vi "LineFollower.vi"() -> ()   [LabVIEW 2019]
uses:
  <vilib>/addons/Fuzzy Logic/TypeDefs/FL System.ctl
  <vilib>/addons/Fuzzy Logic/TypeDefs/FL Variable.ctl
  <vilib>/addons/Fuzzy Logic/TypeDefs/FL Membership Function.ctl
  <vilib>/addons/Fuzzy Logic/TypeDefs/FL Membership Function Shape.ctl
  <vilib>/addons/Fuzzy Logic/TypeDefs/FL Rule.ctl
  <vilib>/addons/Fuzzy Logic/TypeDefs/FL Antecedent.ctl
  <vilib>/addons/Fuzzy Logic/TypeDefs/FL Modifier.ctl
  <vilib>/addons/Fuzzy Logic/TypeDefs/FL Antecedent Connective.ctl
  <vilib>/addons/Fuzzy Logic/TypeDefs/FL Consequent.ctl
  <vilib>/addons/Fuzzy Logic/TypeDefs/FL Consequent Implication.ctl
  <vilib>/addons/Fuzzy Logic/TypeDefs/FL Defuzzification.ctl
  <vilib>/addons/Fuzzy Logic/TypeDefs/FL Interpolating polynomials.ctl
  <vilib>/myRIO/Instrument Drivers/Onboard IO/AI/typedefs/AI Reference.ctl
  <vilib>/myRIO/Common/Instrument Driver Framework/Utilities/typedefs/myRIO Generic Hardware Reference.ctl
  <vilib>/myRIO/Common/Instrument Driver Framework/Utilities/typedefs/Hardware Version Enum.ctl
  <vilib>/myRIO/Common/Instrument Driver Framework/Utilities/typedefs/myRIO v1.0 Reference.ctl
  <vilib>/myRIO/Common/Instrument Driver Framework/Utilities/typedefs/Generic FPGA Reference.ctl
  <vilib>/myRIO/Common/Instrument Driver Framework/myRIO v1.0/AI/typedefs/AI Channels List.ctl
  <vilib>/myRIO/Common/Instrument Driver Framework/myRIO v1.0/AI/typedefs/AI Channels Enum.ctl
  <vilib>/myRIO/Common/Instrument Driver Framework/Utilities/typedefs/Analog Scaling Constants List.ctl
  <vilib>/myRIO/Common/Instrument Driver Framework/Utilities/typedefs/Analog Scaling Constants.ctl
  <vilib>/userdefined/High Color/nirio_resource_hc.ctl
  <vilib>/myRIO/Common/Instrument Driver Framework/Utilities/vis/Is FPGA Ref Available.vi
  <vilib>/myRIO/Common/Instrument Driver Framework/myRIO v1.0/AI/vis/myRIO v1.1 Open AI.vi
  <vilib>/myRIO/Instrument Drivers/Onboard IO/AI/vis/Read.vi
  <vilib>/myRIO/Common/Instrument Driver Framework/Utilities/vis/Validate Channels.vi
  <vilib>/myRIO/Common/Instrument Driver Framework/myRIO v1.0/AI/vis/myRIO v1.0 Reserve AI.vi
  <vilib>/myRIO/Common/Instrument Driver Framework/myRIO v1.0/AI/vis/myRIO v1.0 Build MUX Configuration AI.vi
  <vilib>/myRIO/Common/Instrument Driver Framework/myRIO v1.0/Resource Manager/vis/myRIO v1.0 Reserve Channel List.vi
  <vilib>/myRIO/Common/Instrument Driver Framework/myRIO v1.0/Resource Manager/vis/myRIO v1.0 Reserve Channel.vi
  <vilib>/myRIO/Common/Instrument Driver Framework/myRIO v1.0/Resource Manager/vis/myRIO v1.0 Unreserve Channel.vi
  <vilib>/myRIO/Common/Instrument Driver Framework/myRIO v1.0/Resource Manager/vis/myRIO v1.0 Build Mutex Name.vi
  <vilib>/Utility/VariantDataType/GetNumericInfo.vi
  <vilib>/Utility/error.llb/Error Cluster From Error Code.vi
  <vilib>/myRIO/Common/Instrument Driver Framework/myRIO v1.0/myRIO v1.1 Open.vi
  <vilib>/myRIO/Common/Instrument Driver Framework/myRIO v1.0/AI/vis/myRIO v1.0 Get Scaling Constants AI.vi
  <vilib>/myRIO/Common/Instrument Driver Framework/Utilities/vis/IO Manager.vi
  <vilib>/myRIO/Common/Instrument Driver Framework/Utilities/vis/Configuration Manager.vi
  <vilib>/myRIO/Common/Instrument Driver Framework/myRIO v1.0/myRIO v1.0 Close.vi
  <vilib>/myRIO/Common/Instrument Driver Framework/myRIO v1.0/AI/vis/myRIO v1.0 Read AI.vi
  <vilib>/addons/Fuzzy Logic/FL Fuzzy Controller (MISO).vi
  <vilib>/myRIO/Express VI/Onboard IO/AI/AI Express VI.xnode
  <vilib>/myRIO/Instrument Drivers/Onboard IO/AI/vis/myRIO AI Open.xnode
  <vilib>/myRIO/Instrument Drivers/Onboard IO/AI/AI.lvlib
  <vilib>/addons/Fuzzy Logic/NI_Fuzzy_Logic_API.lvlib
panel:
  out "Zähler Hindernis":i32
  in  "Stop Querstrich":bool
  out "Querstrich/Hindernis detektiert (Output = 1)":dbl
  out "Zeitstempel Fehlermeldung":timestamp
  out "fuzzy system out":T1 {"user MF interpolating polynomials"."coa_x(y) coeff" format="%.4g"; "user MF interpolating polynomials"."Area(y) coeff" format="%.4g"; "user MF interpolating polynomials"."X(y) coeff" format="%.4g"; "user MF interpolating polynomials"."Y(x) coeff" format="%.4g"; "user MF interpolating polynomials"."Y" format="%.4g"; "user MF interpolating polynomials"."X" format="%.4g"; "defuzzification method" items=["Center of Area", "Modified Center of Area", "Center of Sums", "Center of Maximum", "Mean of Maximum"]; "rules"."consequents"."Var Index" min=0; "rules"."consequents"."Cond" items=["=", "!="]; "rules"."consequents"."MF Index" min=0; "rules"."antecedents"."Var Index" min=0; "rules"."antecedents"."Cond" items=["=", "!="]; "rules"."antecedents"."MF Index" min=0; "rules"."consequent implication" items=["Minimum", "Product"]; "rules"."antecedent connective" items=["AND (Minimum)", "AND (Product)", "OR (Maximum)", "OR (Probabilistic)"]; "output variables"."MFs"."shape" items=["Triangle", "Trapezoid", "Singleton", "Sigmoid", "Gaussian", "User-Defined"]; "input variables"."MFs"."shape" items=["Triangle", "Trapezoid", "Singleton", "Sigmoid", "Gaussian", "User-Defined"]}
  out "Fuzzy rule weights":dbl[](array[numeric])
  out "Fuzzy output: Lenkung [-10, 0, 10]":dbl
  out "Input Chart":dbl[](graph)
  out "Input Sensor 1":dbl
  in  "Stop Button":bool
  # "Querstrich / Hindernis Detektion"
  # "Inputs LineFollower"
  # "Outputs LineFollower | Fuzzy-Regelung | Fuzzy Regler muss importiert wird (Line_follower_01.fs)"
  # "IF"
  # "THEN"
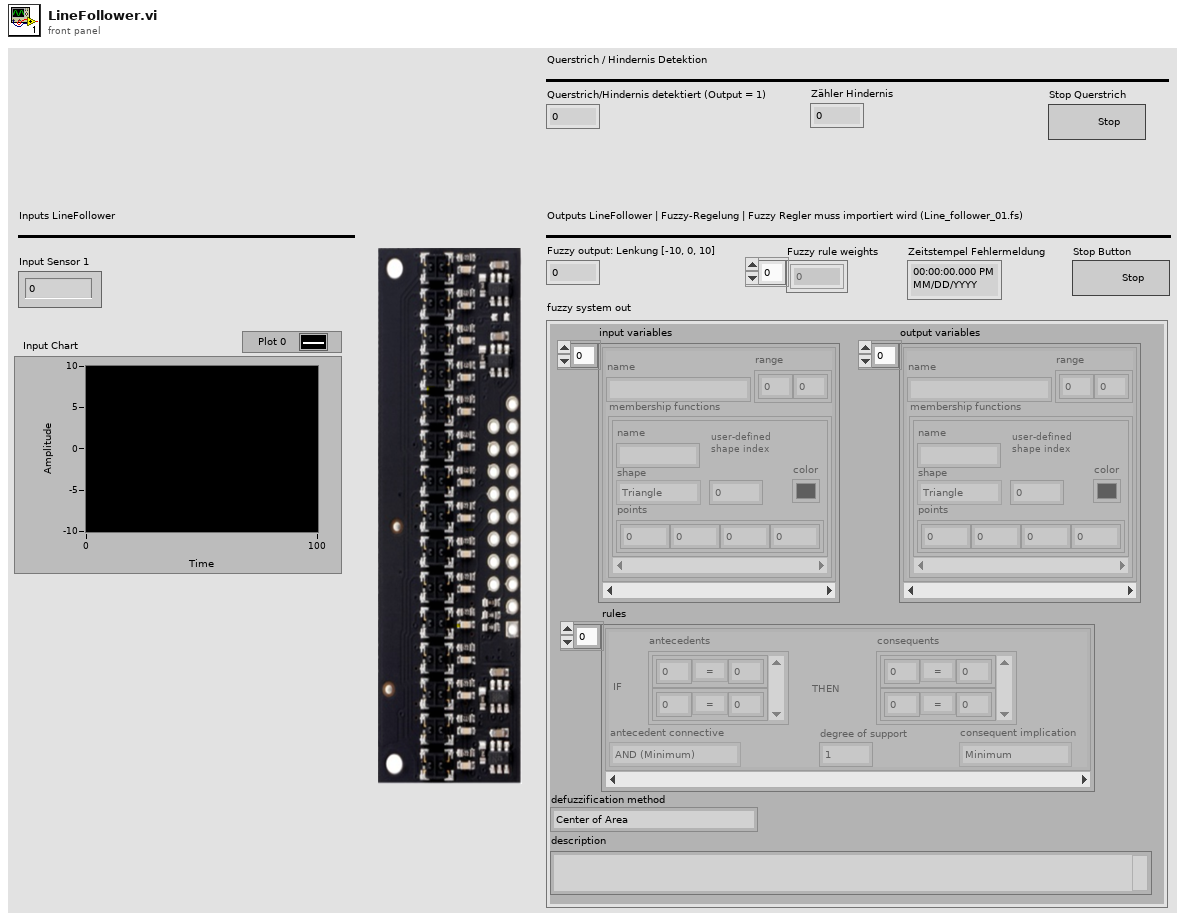
[diagram p1: front panel]
types:
  T1 = typedef "NI_Fuzzy_Logic_API.lvlib/FL System.ctl" = cluster{"input variables":T2[], "output variables":T2[], "rules":T5[], "defuzzification method":T11, "description":string, "user MF interpolating polynomials":T12[]}
  T2 = typedef "NI_Fuzzy_Logic_API.lvlib/FL Variable.ctl" = cluster{"name":string, "range":dbl[], "MFs":T3[]}
  T3 = typedef "NI_Fuzzy_Logic_API.lvlib/FL Membership Function.ctl" = cluster{"name":string, "shape":T4, "points":dbl[], "color":u32, "user-defined shape index":i32}
  T4 = typedef "NI_Fuzzy_Logic_API.lvlib/FL Membership Function Shape.ctl" = u16
  T5 = typedef "NI_Fuzzy_Logic_API.lvlib/FL Rule.ctl" = cluster{"antecedents":T6[], "antecedent connective":T8, "consequents":T9[], "consequent implication":T10, "degree of support":dbl}
  T6 = typedef "NI_Fuzzy_Logic_API.lvlib/FL Antecedent.ctl" = cluster{"Var Index":i32, "MF Index":i32, "Cond":T7}
  T7 = typedef "NI_Fuzzy_Logic_API.lvlib/FL Modifier.ctl" = u16
  T8 = typedef "NI_Fuzzy_Logic_API.lvlib/FL Antecedent Connective.ctl" = u16
  T9 = typedef "NI_Fuzzy_Logic_API.lvlib/FL Consequent.ctl" = cluster{"Var Index":i32, "MF Index":i32, "Cond":T7}
  T10 = typedef "NI_Fuzzy_Logic_API.lvlib/FL Consequent Implication.ctl" = u16
  T11 = typedef "NI_Fuzzy_Logic_API.lvlib/FL Defuzzification.ctl" = u16
  T12 = typedef "NI_Fuzzy_Logic_API.lvlib/FL Interpolating polynomials.ctl" = cluster{"X":dbl[], "Y":dbl[], "Y(x) coeff":dbl[][], "X(y) coeff":dbl[][], "Area(y) coeff":dbl[][], "coa_x(y) coeff":dbl[][]}
  T13 = typedef "AI.lvlib/AI Reference.ctl" = cluster{"myRIO Reference":T14, "AI Channels List":T18, "AI Scaling Constants List":T20}
  T14 = typedef "myRIO Generic Hardware Reference.ctl" = cluster{"myRIO Model":T15, "myRIO Hardware Reference":T16}
  T15 = typedef "Hardware Version Enum.ctl" = enum16{"Unknown", "myRIO-1900", "myRIO-1950", "roboRIO", "NI ELVIS RIO CM", "ELVIS III"}
  T16 = typedef "myRIO v1.0 Reference.ctl" = cluster{"Generic FPGA Reference":T17, "Allow multiple opens":bool}
  T17 = typedef "Generic FPGA Reference.ctl" = refnum<k20>
  T18 = typedef "AI Channels List.ctl" = T19[]
  T19 = typedef "AI Channels Enum.ctl" = enum16{"Not Connected", "AudioIn/Left", "AudioIn/Right", "C/AI0", "C/AI1", "A/AI0", "A/AI1", "A/AI2", "A/AI3", "A/AI4", "A/AI5", "A/AI6", "A/AI7", "B/AI0", "B/AI1", "B/AI2", "B/AI3", "B/AI4", "B/AI5", "B/AI6", "B/AI7", "AI/AI0", "AI/AI1", "AI/AI2", "AI/AI3", "A/AI0 (DIFF)", "A/AI1 (DIFF)", "A/AI2 (DIFF)", "A/AI3 (DIFF)", "B/AI0 (DIFF)", "B/AI1 (DIFF)", "B/AI2 (DIFF)", "B/AI3 (DIFF)"}
  T20 = typedef "Analog Scaling Constants List.ctl" = T21[]
  T21 = typedef "Analog Scaling Constants.ctl" = cluster{"LSB Weight (Volts)":dbl, "Offset (Volts)":dbl, "Signed?":bool}
  T22 = typedef "nirio_resource_hc.ctl" = tag
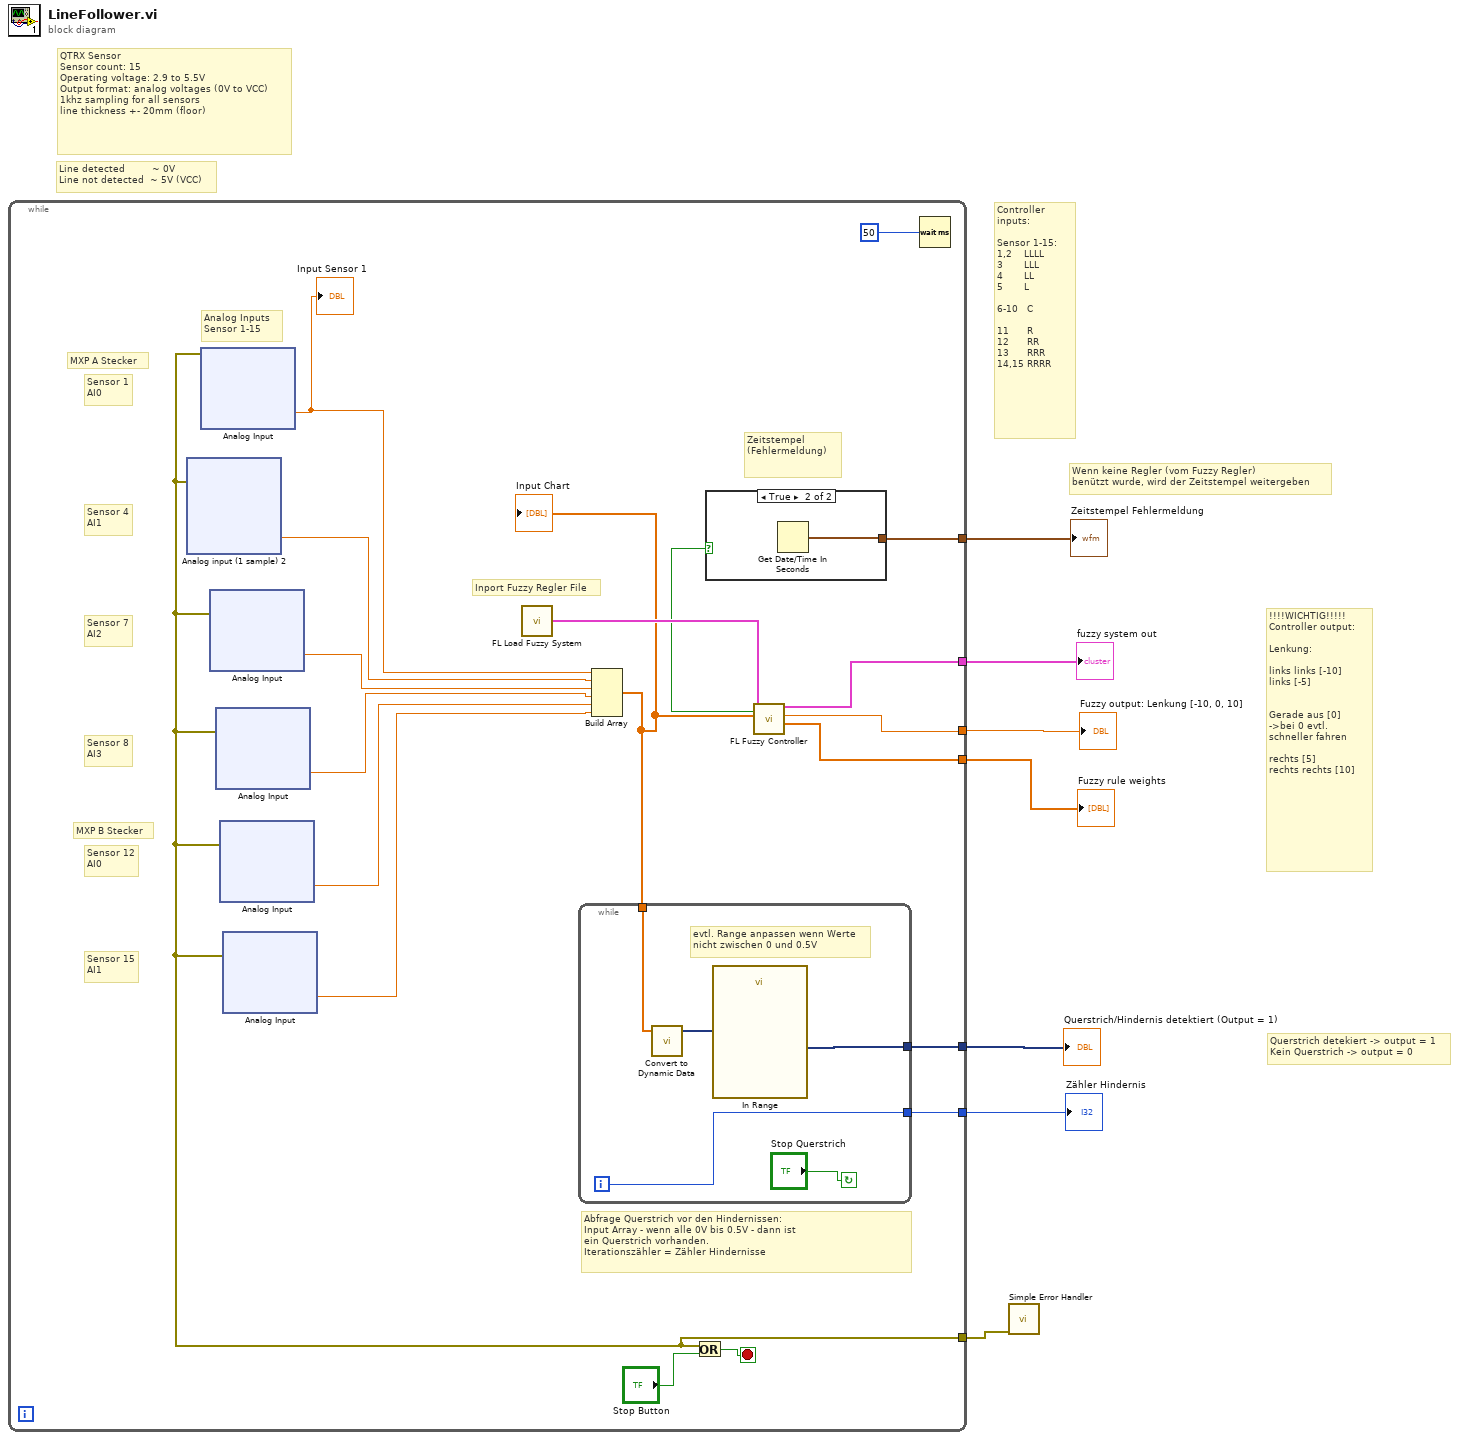
[diagram p0: block diagram]
diagram:
  # "Querstrich detekiert -> output = 1\nKein Querstrich -> output = 0"
  # "Controller inputs:\n\nSensor 1-15:\n1,2    LLLL\n3       LLL\n4       LL\n5       L\n\n6-10   C\n\n11      R\n12      RR\n13      RRR\n14,15 RRRR"
  # "!!!!WICHTIG!!!!!\nController output:\n\nLenkung:\n\nlinks links [-10]\nlinks [-5]\n\n\nGerade aus [0]\n->bei 0 evtl. schneller fahren \n\nrechts [5]\nrechts rechts [10]"
  # "Wenn keine Regler (vom Fuzzy Regler)\nbenützt wurde, wird der Zeitstempel weitergeben"
  # "Line detected         ~ 0V \nLine not detected  ~ 5V (VCC)"
  # "QTRX Sensor\nSensor count: 15\nOperating voltage: 2.9 to 5.5V\nOutput format: analog voltages (0V to VCC)\n1khz sampling for all sensors\nline thickness +- 20mm (floor)"
  n1 = while {
    tunnel: [w13] -> w7
    tunnel: [w19] -> w6
    tunnel: [w22] -> w5
    tunnel: [w21] -> w4
    tunnel: [w18] -> w3
    tunnel: [w16] -> w2
    tunnel: [w15] -> w1
    stop <- w24 stop-if-true
    # "MXP B Stecker"
    # "MXP A Stecker"
    # "Sensor 15\nAI1"
    # "Sensor 8\nAI3"
    # "Sensor 7\nAI2"
    # "Sensor 12\nAI0"
    # "Sensor 4\nAI1"
    # "Sensor 1\nAI0"
    # "Abfrage Querstrich vor den Hindernissen:\nInput Array - wenn alle 0V bis 0.5V - dann ist\nein Querstrich vorhanden.\nIterationszähler = Zähler Hindernisse"
    # "Zeitstempel (Fehlermeldung)"
    # "Inport Fuzzy Regler File"
    # "Analog Inputs \nSensor 1-15"
    n2 = xnode ("Analog Input")() -> ("A/AI0 (Pin 3)"=w14:dbl, "error out"=w13:errorcluster)  [unwired: 1 in]
    "Input Sensor 1" <- w14
    n3 = xnode "Analog input (1 sample) 2"("error in (no error)"=w13) -> ("A/AI1 (Pin 5)"=w12:dbl)  [unwired: 1 out]
    n4 = xnode ("Analog Input")("error in (no error)"=w13) -> ("A/AI2 (Pin 7)"=w11:dbl)  [unwired: 1 out]
    n5 = xnode ("Analog Input")("error in (no error)"=w13) -> ("A/AI3 (Pin 9)"=w10:dbl)  [unwired: 1 out]
    n6 = xnode ("Analog Input")("error in (no error)"=w13) -> ("B/AI0 (Pin 3)"=w9:dbl)  [unwired: 1 out]
    n7 = xnode ("Analog Input")("error in (no error)"=w13) -> ("B/AI1 (Pin 5)"=w8:dbl)  [unwired: 1 out]
    n8 = call <vilib>:"FL Load Fuzzy System.vi"() -> ("fuzzy system out"=w23:T1)  [unwired: 10 in, 1 out]
    n9 = Build Array(w14, w12, w11, w10, w9, w8) -> (w17:dbl[])
    "Input Chart" <- w17
    n10 = while {
      tunnel: w17 -> [w68]
      tunnel: [w66] -> w16
      tunnel: [w64] -> w15
      i -> [w64]
      stop <- "Stop Querstrich" continue-if-true
      # "evtl. Range anpassen wenn Werte\nnicht zwischen 0 und 0.5V"
      n11 = call "Convert to Dynamic Data"("Array"=w68) -> ("Dynamic Data Type"=w67:dynamicdata)  [unwired: 3 in]
      n12 = call "In Range"("Operand 1"=w67) -> ("Result"=w66:dynamicdata)  [unwired: 9 in, 1 out]
    }
    n13 = Or(x=w13, y="Stop Button") -> (x .or. y?=w24:bool)
    n14 = call-poly <vilib>:"FL Fuzzy Controller.vi"("input values"=w17, "fuzzy system in"=w23) -> ("rule weights"=w22:dbl[], "output value"=w19:dbl, "fuzzy system out"=w21:T1, "rule-invoked value?"=w20:bool)  [unwired: 5 in, 1 out]
    n15 = case shown="True" w20 {
      tunnel: [_ w69] -> w18
      frame False {
      }
      frame True {
        n16 = Get Date/Time In Seconds() -> (seconds since 1Jan1904=w69:timestamp)
      }
    }
    n17 = Wait (ms)(milliseconds to wait=50) -> ()  [unwired: 1 out]
  }
  "Fuzzy output: Lenkung [-10, 0, 10]" <- w6
  "Fuzzy rule weights" <- w5
  "fuzzy system out" <- w4
  "Zeitstempel Fehlermeldung" <- w3
  "Querstrich/Hindernis detektiert (Output = 1)" <- w2
  "Zähler Hindernis" <- w1
  n18 = call <vilib>:"Simple Error Handler.vi"("error in (no error)"=w7) -> ()  [unwired: 4 in, 5 out]
